vi "JSON parser.vi"(10 "JSON string":string="{\r\n  \"incoming typed relationships\"  : \"http://localhost:9999/node/8/relationships/in/{-list|&|types}\",\r\n  \"incoming relationships\" : \"http://localhost:9999/node/8/relationships/in\",\r\n  \"all relationships\" : \"http://localhost:9999/node/8/relationships/all\",\r\n  \"create relationship\" : \"http://localhost:9999/node/8/relationships\",\r\n  \"data\" : {\r\n    \"Name\" : \"Product 808\",\r\n    \"Number\" : 808\n\r  },\r\n  \"traverse\" : \"http://localhost:9999/node/8/traverse/{returnType}\",\r\n  \"property\" : \"http://localhost:9999/node/8/properties/{key}\",\r\n  \"self\" : \"http://localhost:9999/node/8\",\r\n  \"properties\" : \"http://localhost:9999/node/8/properties\",\r\n  \"all typed relationships\" : \"http://localhost:9999/node/8/relationships/all/{-list|&|types}\",\r\n  \"outgoing typed relationships\" : \"http://localhost:9999/node/8/relationships/out/{-list|&|types}\",\r\n  \"outgoing relationships\" : \"http://localhost:9999/node/8/relationships/out\"\r\n}") -> (1 "values":string[](array[string]), 2 "keys":string[](array[string]))   [LabVIEW 2011]
panel:
  out "result string":string
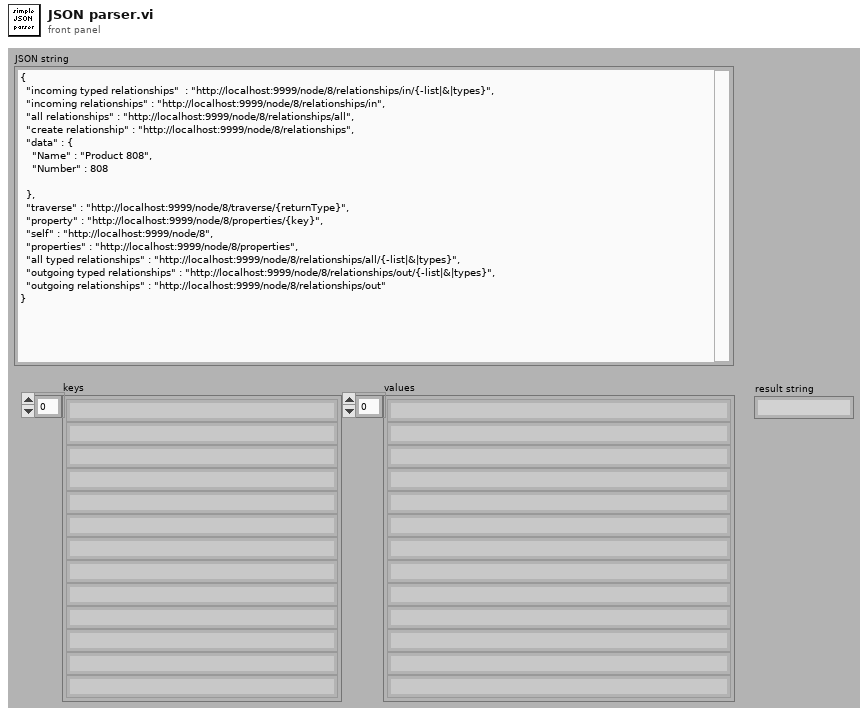
[diagram p1: front panel]
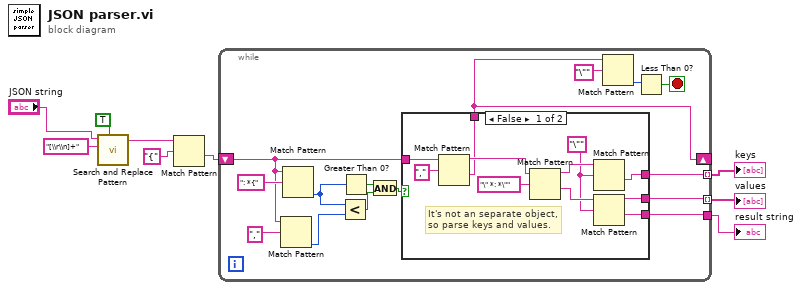
[diagram p0: block diagram]
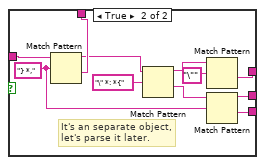
[diagram p2: hidden frame]
diagram:
  n1 = call <vilib>:"Search and Replace Pattern.vi"("string"="JSON string", "regular expression (\"\")"="[\\r\\n]+" ("regular expression (\"\")"), "replace all? (F)"=TRUE) -> ("result string"=w8:string)  [unwired: 2 in, 1 out]
  n2 = Match Pattern(string=w8, regular expression="{" ("search string/char (-)")) -> (after substring=w5:string)  [unwired: 1 in, 3 out]
  n3 = while {
    tunnel: [w21] -> w4 mode=indexing
    tunnel: [w20] -> w3 mode=indexing
    shift-right: [w17] -> _
    shift-left: w5 -> [w15]
    tunnel: [w19] -> w2
    stop <- w22 stop-if-true
    n4 = Match Pattern(string=w15, regular expression="," ("search string/char (-)")) -> (offset past match=w14:i32)  [unwired: 1 in, 3 out]
    n5 = Match Pattern(string=w15, regular expression=": *{") -> (offset past match=w13:i32)  [unwired: 1 in, 3 out]
    n6 = Less?(x=w13, y=w14) -> (x < y?=w11:bool)
    n7 = Greater Than 0?(x=w13) -> (x > 0?=w12:bool)
    n8 = And(x=w12, y=w11) -> (x .and. y?=w10:bool)
    n9 = case shown="False" w10 {
      tunnel: [w31 w42] -> w21
      tunnel: [w30 w41] -> w20
      tunnel: [w29 w40] -> w19
      tunnel: w15 -> [w27 w39]
      tunnel: [w25 w38] -> w17
      frame False {
        w32 = "\"" ("regular expression")
        # "It's not an separate object,\nso parse keys and values."
        n10 = Match Pattern(string=w27, regular expression="," ("search string/char (-)")) -> (before substring=w26:string, after substring=w25:string)  [unwired: 1 in, 2 out]
        n11 = Match Pattern(string=w26, regular expression="\" *: *\"") -> (before substring=w34:string, after substring=w33:string)  [unwired: 1 in, 2 out]
        n12 = Match Pattern(string=w34, regular expression=w32) -> (after substring=w31:string)  [unwired: 1 in, 3 out]
        n13 = Match Pattern(string=w33, regular expression=w32) -> (before substring=w30:string, after substring=w29:string)  [unwired: 1 in, 2 out]
      }
      frame True {
        w36 = "} *," ("search string/char (-)")
        # "It's an separate object,\nlet's parse it later."
        n14 = Match Pattern(string=w39, regular expression=w36) -> (before substring=w37:string, after substring=w38:string)  [unwired: 1 in, 2 out]
        n15 = Match Pattern(string=w37, regular expression="\" *: *{") -> (before substring=w45:string, after substring=w44:string)  [unwired: 1 in, 2 out]
        n16 = Match Pattern(string=w45, regular expression="\"") -> (after substring=w42:string)  [unwired: 1 in, 3 out]
        n17 = Match Pattern(string=w44, regular expression=w36) -> (before substring=w41:string, after substring=w40:string)  [unwired: 1 in, 2 out]
      }
    }
    n18 = Match Pattern(string=w17, regular expression="\"" ("search string/char (-)")) -> (offset past match=w23:i32)  [unwired: 1 in, 3 out]
    n19 = Less Than 0?(x=w23) -> (x < 0?=w22:bool)
  }
  "keys" <- w4
  "values" <- w3
  "result string" <- w2
